vi "Auto-fit xyscan-single data_YCC.vi"() -> ()   [LabVIEW 2014]
uses:
  <vilib>/Analysis/6fits.llb/Curve Fitting Criteria.ctl
  <vilib>/Utility/file.llb/Read From Spreadsheet File (DBL).vi
  <vilib>/Analysis/polynomials.llb/1D Polynomial Evaluation (DBL).vi
  <vilib>/gmath/NumericalOptimization/Nonlinear Curve Fit LM formula string.vi
  <vilib>/Analysis/NI_AALPro.lvlib
  <vilib>/gmath/NI_Gmath.lvlib
panel:
  in  "termination":cluster{"max iteration":i32, "tolerance":dbl}={"max iteration"=200, "tolerance"=1e-08}
  out "XY Graph 2":cluster{dbl[], dbl[]}(graph)
  in  "OK to fit?":bool
  in  "initial parameters":dbl[](array[numeric])=[-3.5, 12.7, 0.6, 0.2]
  out "best fit parameters":dbl[](array[numeric])
  in  "Gaussian fit?":bool
  out "Stage":dbl[](array[numeric])
  out "QPD":dbl[](array[numeric])
  out "Polynomial Coefficients":dbl[](array[numeric])
  in  "polynomial order":i32=1
  in  "stop":bool
  out "XY Graph":cluster{"all rows":dbl[], "all rows":dbl[]}[](graph)
  in  "X=T\nY=F":bool
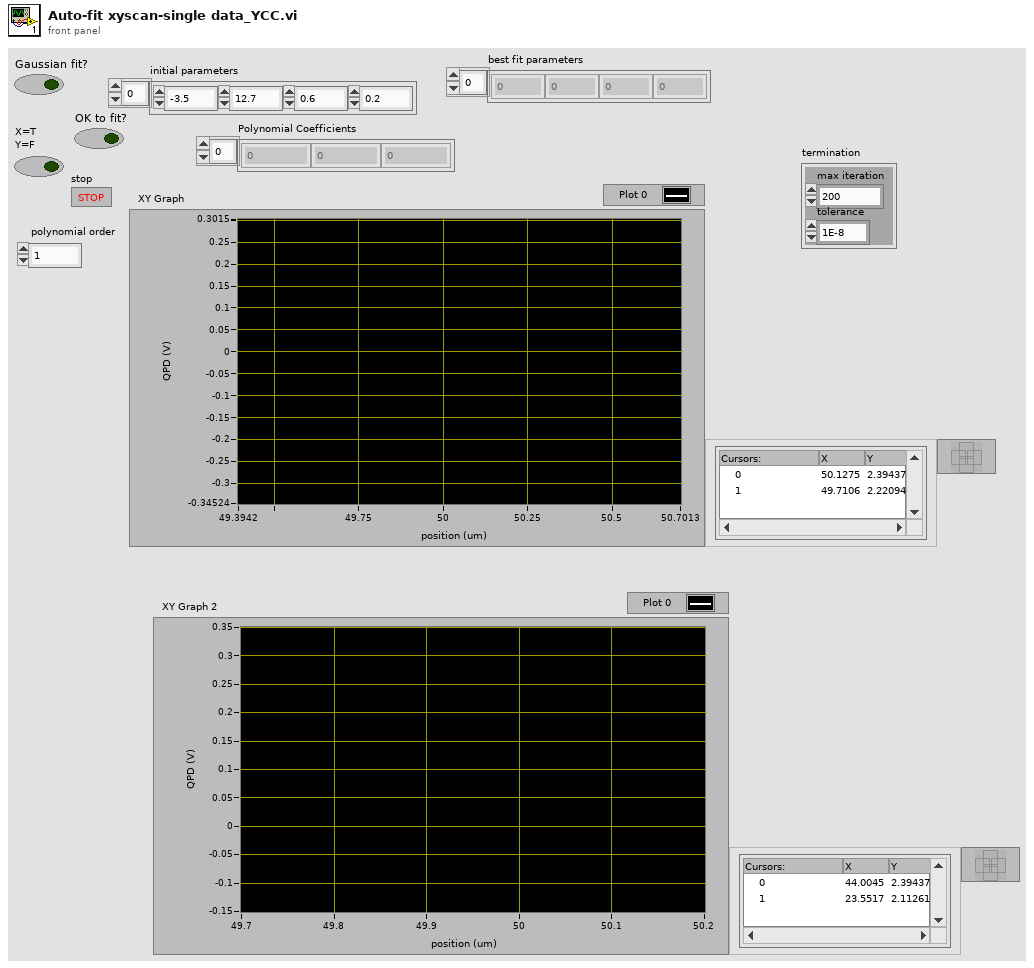
[diagram p1: front panel]
types:
  T1 = cluster{"model":string, "Parameters":string[], "x":string}
  T2 = typedef "NI_AALPro.lvlib/Curve Fitting Criteria.ctl" = u16
  T3 = cluster{"all rows":dbl[], "best nonlinear fit":dbl[]}[]
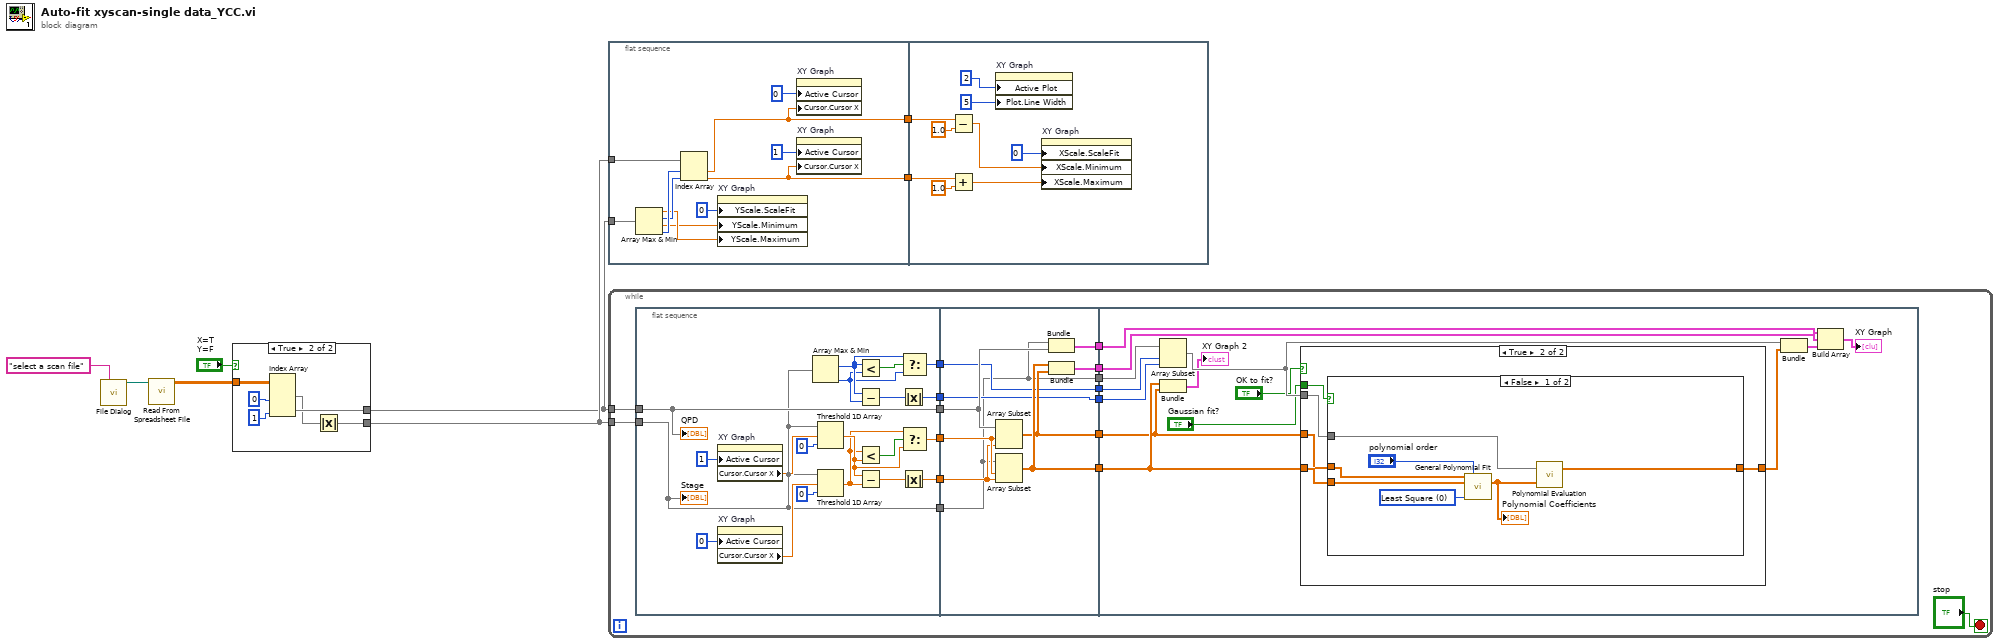
[diagram p0: block diagram]
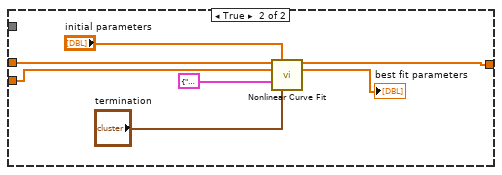
[diagram p3: hidden frame]
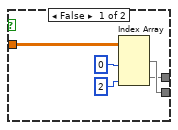
[diagram p4: hidden frame]
diagram:
  n1 = call "File Dialog"("prompt"="select a scan file") -> ("selected path"=w7:path)  [unwired: 11 in, 3 out]
  n2 = call-poly <vilib>:"Read From Spreadsheet File.vi"("file path (dialog if empty)"=w7) -> ("all rows"=w6:dbl[][])  [unwired: 6 in, 4 out]
  n3 = case shown="True" "X=T\nY=F" {
    tunnel: w6 -> [w11 w19]
    tunnel: [w10 w14] -> w4
    tunnel: [w9 w16] -> w3
    frame False {
      n4 = Index Array(array=w11, index (col) #1=0 ("disabled index (col)"), index (col) #2=2 ("index (col)")) -> (element #1=w10:dbl[], element #2=w9:dbl[])  [unwired: 2 in]
    }
    frame True {
      n5 = Index Array(array=w19, index (col) #1=0 ("disabled index (col)"), index (col) #2=1 ("index (col)")) -> (element #1=w15:dbl[], element #2=w16:dbl[])  [unwired: 2 in]
      n6 = Absolute Value(x=w15) -> (abs(x)=w14:dbl[])
    }
  }
  n7 = flat-sequence {
    tunnel: w4 -> [w27]
    tunnel: w3 -> [w28]
    tunnel: [w24] -> w2
    tunnel: [w23] -> w1
    tunnel: w2 -> [w36]
    tunnel: w1 -> [w34]
    frame #0 {
      n8 = Array Max & Min(array=w28) -> (max value=w21:dbl, max index (indices)=w25:i32, min value=w20:dbl, min index (indices)=w26:i32)
      n9 = Index Array(array=w27, index #1=w26, index #2=w25) -> (element #1=w24:dbl, element #2=w23:dbl)
      n10 = property on="XY Graph" class="XYGraph (strict)"("YScale.ScaleFit"=u8 0 ("Y Scale.Scale Fit"), "YScale.Minimum"=w20, "YScale.Maximum"=w21) -> ()  [unwired: 2 in, 2 out]
      n11 = property on="XY Graph" class="XYGraph (strict)"("Active Cursor"=u32 0, "Cursor.Cursor X"=w24) -> ()  [unwired: 2 in, 2 out]
      n12 = property on="XY Graph" class="XYGraph (strict)"("Active Cursor"=u32 1, "Cursor.Cursor X"=w23) -> ()  [unwired: 2 in, 2 out]
    }
    frame #1 {
      n13 = Subtract(x=w36, y=1.0) -> (x-y=w32:dbl)
      n14 = Add(x=w34, y=1.0) -> (x+y=w31:dbl)
      n15 = property on="XY Graph" class="XYGraph (strict)"("Active Plot"=u32 2, "Plot.Line Width"=u8 5) -> ()  [unwired: 2 in, 2 out]
      n16 = property on="XY Graph" class="XYGraph (strict)"("XScale.ScaleFit"=u8 0 ("X Scale.Scale Fit"), "XScale.Minimum"=w32, "XScale.Maximum"=w31) -> ()  [unwired: 2 in, 2 out]
    }
  }
  n17 = while {
    tunnel: w4 -> [w55]
    tunnel: w3 -> [w52]
    stop <- "stop" stop-if-true
    n18 = flat-sequence {
      tunnel: w55 -> [w68]
      tunnel: [w68] -> w54
      tunnel: [w71] -> w53
      tunnel: w52 -> [w71]
      tunnel: [w56] -> w51
      tunnel: [w60] -> w50
      tunnel: [w66] -> w45
      tunnel: [w62] -> w43
      tunnel: w54 -> [w78]
      tunnel: w53 -> [w83]
      tunnel: w51 -> [w85]
      tunnel: w50 -> [w84]
      tunnel: [w82] -> w48
      tunnel: [w81] -> w47
      tunnel: [w80] -> w46
      tunnel: w45 -> [w80]
      tunnel: [w79] -> w44
      tunnel: w43 -> [w79]
      tunnel: [w78] -> w42
      tunnel: [w77] -> w41
      tunnel: [w76] -> w40
      tunnel: w48 -> [w88]
      tunnel: w47 -> [w86]
      tunnel: w46 -> [w99]
      tunnel: w44 -> [w98]
      tunnel: w42 -> [w97]
      tunnel: w41 -> [w93]
      tunnel: w40 -> [w92]
      frame #0 {
        n19 = property on="XY Graph" class="XYGraph (strict)"("Active Cursor"=u32 1) -> ("Cursor.Cursor X"=w69:dbl)  [unwired: 2 in, 2 out]
        n20 = property on="XY Graph" class="XYGraph (strict)"("Active Cursor"=u32 0) -> ("Cursor.Cursor X"=w70:dbl)  [unwired: 2 in, 2 out]
        n21 = Array Max & Min(array=w68) -> (max index (indices)=w64:i32, min index (indices)=w63:i32)  [unwired: 2 out]
        n22 = Threshold 1D Array(1:0 ("start index (0)"), 2:w69, 3:w68) -> (0:w58:dbl)
        n23 = Threshold 1D Array(1:0 ("start index (0)"), 2:w70, 3:w68) -> (0:w57:dbl)
        n24 = Less?(x=w64, y=w63) -> (x < y?=w65:bool)
        n25 = Subtract(x=w64, y=w63) -> (x-y=w67:i32)
        n26 = Less?(x=w57, y=w58) -> (x < y?=w59:bool)
        n27 = Subtract(x=w58, y=w57) -> (x-y=w61:dbl)
        n28 = Absolute Value(x=w67) -> (abs(x)=w66:i32)
        n29 = Absolute Value(x=w61) -> (abs(x)=w60:dbl)
        n30 = Select(t=w64, s=w65, f=w63) -> (s? t:f=w62:i32)
        n31 = Select(t=w57, s=w59, f=w58) -> (s? t:f=w56:dbl)
        "QPD" <- w71
        "Stage" <- w68
      }
      frame #1 {
        n32 = Array Subset(array=w83, index=w85, length=w84) -> (w81:dbl[])
        n33 = Array Subset(array=w78, index=w85, length=w84) -> (w82:dbl[])
        n34 = Bundle("all rows"=w78, "all rows"=w83) -> (w77:cluster{"all rows":dbl[], "all rows":dbl[]})  [unwired: 1 in]
        n35 = Bundle(w82, w81) -> (w76:cluster{dbl[], dbl[]})  [unwired: 1 in]
      }
      frame #2 {
        n36 = Array Subset(array=w97, index=w98, length=w99) -> (w96:dbl[])
        n37 = Bundle(w88, w86) -> (→"XY Graph 2":cluster{dbl[], dbl[]})  [unwired: 1 in]
        n38 = case shown="True" "OK to fit?" {
          tunnel: w88 -> [w100 w105]
          tunnel: w86 -> [_ w104]
          tunnel: w96 -> [_ w103]
          tunnel: [w100 w102] -> w95
          tunnel: "Gaussian fit?" -> [_ w101]
          frame False {
          }
          frame True {
            n39 = case shown="False" w101 {
              tunnel: w105 -> [w111 w115]
              tunnel: w104 -> [w110 w113]
              tunnel: w103 -> [w108 _]
              tunnel: [w107 w118] -> w102
              frame False {
                w109 = T2 0 items=["Least Square", "Least Absolute Residual", "Bisquare"] ("method")
                n40 = call <vilib>:"General Polynomial Fit.vi"("Y"=w110, "polynomial order"="polynomial order", "X"=w111, "method"=w109) -> ("Polynomial Coefficients"=w106:dbl[])  [unwired: 8 in, 3 out]
                "Polynomial Coefficients" <- w106
                n41 = call-poly <vilib>:"Polynomial Evaluation.vi"("P(x)"=w106, "A"=w108) -> ("P(A)"=w107:dbl[])  [unwired: 1 out]
              }
              frame True {
                n42 = call-poly <vilib>:"Nonlinear Curve Fit.vi"("Y"=w113, "initial parameters"="initial parameters", "X"=w115, "model description"=T1 {"model"="a1*(u-a2)*exp((-(u-a2)^2)/(a3^2))+a4", "Parameters"=["a1", "a2", "a3", "a4"], "x"="u"}, "termination"="termination") -> ("best nonlinear fit"=w118:dbl[], "best fit parameters"=→"best fit parameters":dbl[])  [unwired: 6 in, 3 out]
              }
            }
          }
        }
        n43 = Bundle(w96, "best nonlinear fit"=w95) -> (w94:cluster{dbl[], "best nonlinear fit":dbl[]})  [unwired: 1 in]
        n44 = Build Array(w93, w92, w94) -> (→"XY Graph":T3)
      }
    }
  }
